vi "Configure Averaging.vi"(0 "VISA resource name":refnum<visa-resource-name>, 1 "Auto Averaging (T: Enable)":bool=TRUE, 5 "Channel (1: Channel A)":u16(ring)=1 items=["Channel A"=1, "Channel B"=2], 7 "Averaging Count (4)":i32=4, 11 "error in (no error)":errorcluster) -> (4 "VISA resource name out":refnum<visa-resource-name>, 15 "error out":errorcluster)   [LabVIEW 2013, in "Template - Power Meter.lvlib"]
doc: "Configure the settings which dictate how the average of the measurements is calculated."
uses:
  <instrlib>/_Template - Power Meter/Template - Power Meter.lvlib
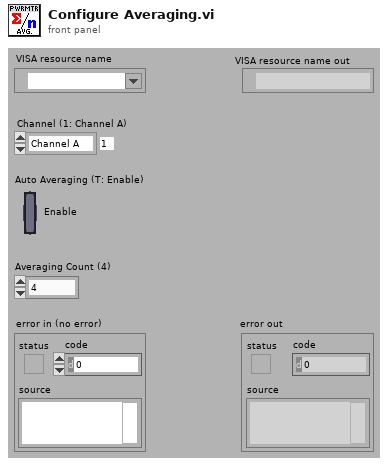
[diagram p1: front panel]
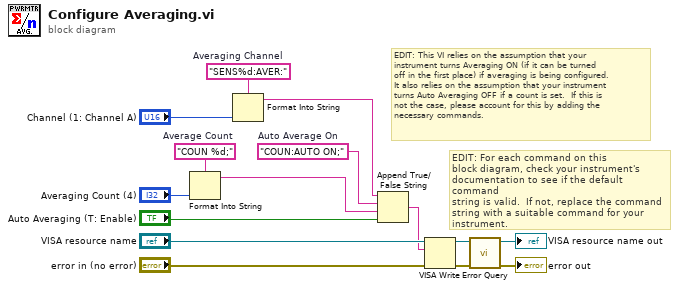
[diagram p0: block diagram]
diagram:
  w4 = "COUN:AUTO ON;"  # Auto Average On
  w7 = "COUN %d;"  # Average Count
  w8 = "SENS%d:AVER:"  # Averaging Channel
  # "EDIT: This VI relies on the assumption that your\ninstrument turns Averaging ON (if it can be turned \noff in the first place) if averaging is being configured.\nIt also relies on the assumption that your instrument\nturns Auto Averaging OFF if a count is set.  If this is\nnot the case, please account for this by adding the\nnecessary commands."
  # "EDIT: For each command on this\nblock diagram, check your instrument's\ndocumentation to see if the default command\nstring is valid.  If not, replace the command\nstring with a suitable command for your\ninstrument."
  n1 = Format Into String(format string=w7, "Averaging Count (4)") -> (resulting string=w9:string)  [unwired: 2 in, 1 out]
  n2 = Format Into String(format string=w8, "Channel (1: Channel A)") -> (resulting string=w5:string)  [unwired: 2 in, 1 out]
  n3 = Append True/False String(1:"Auto Averaging (T: Enable)", 2:w9, 3:w4, 4:w5) -> (0:w3:string)
  n4 = VISA Write(VISA resource name="VISA resource name", write buffer=w3, error in (no error)="error in (no error)") -> (VISA resource name out=w13:refnum<visa-resource-name>, error out=w11:errorcluster)  [unwired: 1 out]
  n5 = call <instrlib>:"Error Query.vi"("error in (no error)"=w11, "VISA resource name"=w13) -> ("error out"=→"error out":errorcluster, "VISA resource name out"=→"VISA resource name out":refnum<visa-resource-name>)  [unwired: 6 in, 2 out]
